vi "AUTO - REVERSE from DASHB.vi"() -> ()   [LabVIEW 2020]
uses:
  Robot Global Data.vi
  <vilib>/Rock Robotics/Network Tables/NT Write Boolean.vi
  <vilib>/Rock Robotics/WPI/Utilities/WPI_GetSetVariantRefNum.vi
  <vilib>/Rock Robotics/Network Tables/NT Read Number.vi
  <vilib>/Rock Robotics/Network Tables/NT Read Boolean.vi
  <vilib>/Rock Robotics/Network Tables/NT Write Number.vi
panel:
  out "time drive (s)":dbl
  out "SHOOTER %PREV":dbl
  in  "NT stack ref":string="AUTO SET/"
  out "motor command":dbl
  out "motor run time (s)":dbl
  out "distance (in)":dbl
  out "free velocity (in/s)":dbl
  out "throttle":dbl
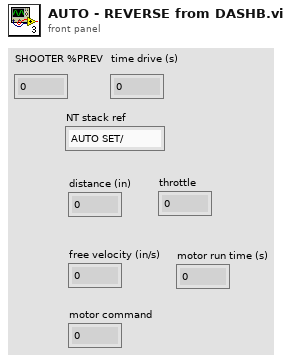
[diagram p1: front panel]
types:
  T1 = cluster{"DRIVE gear ratio":dbl, "DRIVE wheel diameter (in)":dbl, "DRIVE free speed rpm":dbl, "DRIVE min output":dbl, "DRIVE stall in-lbf":dbl}
  T2 = typedef "WPI_RobotDriveDevRef.ctl" = cluster{"DevStatus":errorcluster, "Motors[]":T3[], "Square Inputs":bool, "Max Output":dbl}
  T3 = typedef "WPI_MotorControlDeviceRef.ctl" = cluster{"DeviceStatus":errorcluster, "Type":T4, "PWM":cluster{"PWM Channel":T5, "DeadBand":T6}, "CAN":cluster{"Device Number":u8, "SetOutput VI Ref":variant, "GetOutput VI Ref":variant, "Enable VI Ref":variant, "Disable VI Ref":variant, "Data":variant}, "Invert":bool, "DIO PWM":cluster{"PWM \"Enable\" Channel":T5, "DIOChannel":T7, "PWM Rate":dbl}}
  T4 = typedef "WPI_MotorControlType.ctl" = enum16{"PWM", "CAN", "DIO PWM"}
  T5 = typedef "FPGA_DIOPWMChannel.ctl" = enum8{"PWM 0", "PWM 1", "PWM 2", "PWM 3", "PWM 4", "PWM 5", "PWM 6", "PWM 7", "PWM 8", "PWM 9", "PWM MXP 0", "PWM MXP 1", "PWM MXP 2", "PWM MXP 3", "PWM MXP 4", "PWM MXP 5", "PWM MXP 6", "PWM MXP 7", "PWM MXP 8", "PWM MXP 9", "Invalid"}
  T6 = typedef "WPI_PWMDeadband.ctl" = cluster{"Name":string, "maxPositivePwm":i32, "minPositivePwm":i32, "centerPwm":i32, "maxNegativePwm":i32, "minNegativePwm":i32, "angularRange":u16}
  T7 = typedef "FPGA_DIOChannel.ctl" = enum8{"DIO 0", "DIO 1", "DIO 2", "DIO 3", "DIO 4", "DIO 5", "DIO 6", "DIO 7", "DIO 8", "DIO 9", "DIO MXP 0", "DIO MXP 1", "DIO MXP 2", "DIO MXP 3", "DIO MXP 4", "DIO MXP 5", "DIO MXP 6", "DIO MXP 7", "DIO MXP 8", "DIO MXP 9", "DIO MXP 10", "DIO MXP 11", "DIO MXP 12", "DIO MXP 13", "DIO MXP 14", "DIO MXP 15", "SPI Port CS1", "SPI Port CS2", "SPI Port CS3", "SPI Port MISO", "SPI Port MOSI", "Invalid"}
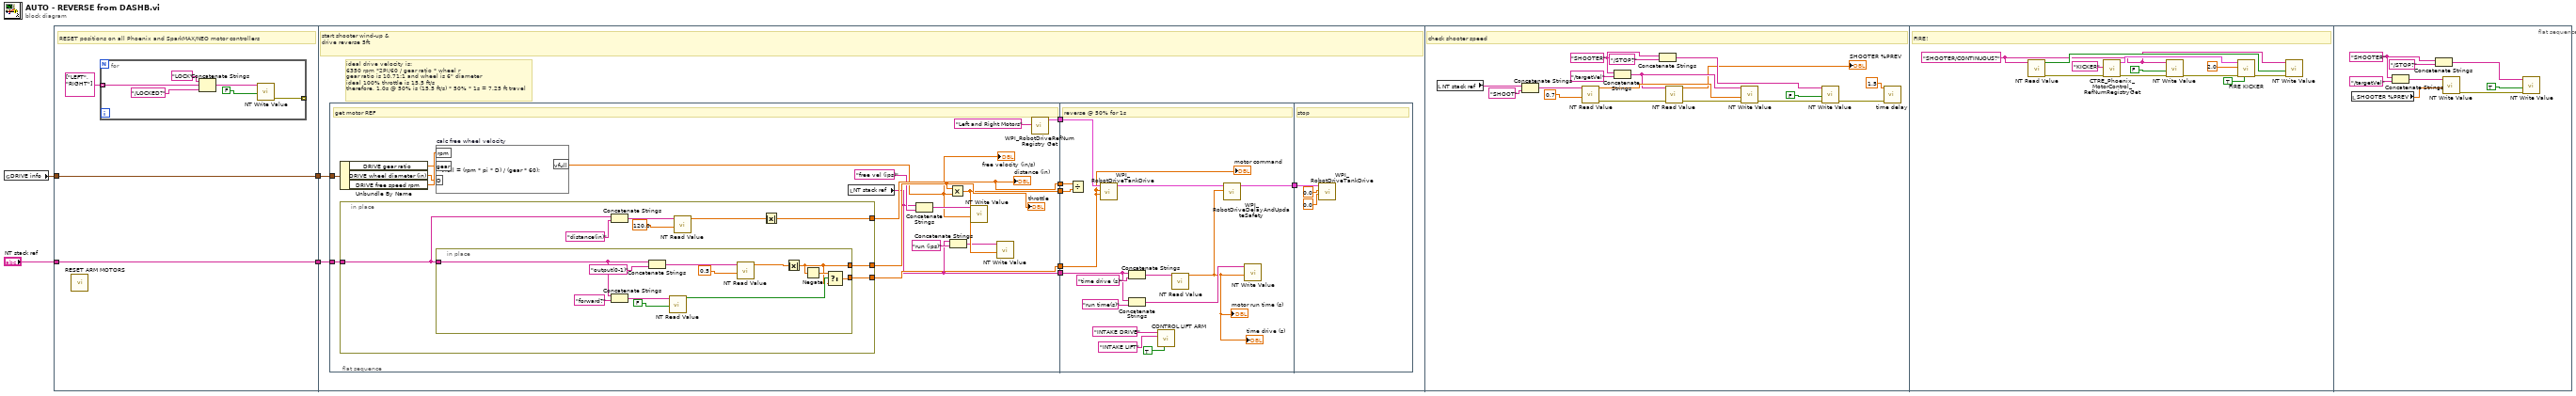
[diagram p0: block diagram]
diagram:
  n1 = global read "Robot Global Data.vi" "DRIVE info"() -> (w4:T1)
  n2 = flat-sequence {
    tunnel: w4 -> [w6]
    tunnel: [w6] -> w2
    tunnel: "NT stack ref" -> [w5]
    tunnel: [w5] -> w1
    tunnel: w2 -> [w15]
    tunnel: w1 -> [w14]
    frame #0 {
      # "RESET positions on all Phoenix and SparkMAX/NEO motor controllers"
      n3 = call "RESET ARM MOTORS.vi"() -> ()  [unwired: 9 in, 3 out]
      n4 = for {
        tunnel: string[] ["LEFT", "RIGHT"] -> [w10] mode=indexing
        tunnel: [w8] -> _ mode=indexing
        n5 = Concatenate Strings("LOCK" ("string"), w10, "/LOCKED?" ("Name")) -> (w12:string)
        n6 = call-poly <vilib>:"NT Write Value.vi"("Boolean"=FALSE, "Name"=w12) -> ("error out"=w8:errorcluster)  [unwired: 9 in]
      }
    }
    frame #1 {
      # "ideal drive velocity is:\n6350 rpm *2PI/60 / gear ratio * wheel r\ngear ratio is 10.71:1 and wheel is 6\" diameter\nideal 100% throttle is 15.5 ft/s\ntherefore, 1.0s @ 50% is (15.5 ft/s) * 50% * 1s = 7.25 ft travel"
      # "start shooter wind-up &\ndrive reverse 5ft"
      n7 = flat-sequence {
        tunnel: [w37] -> w21
        tunnel: w15 -> [w36]
        tunnel: w14 -> [w32]
        tunnel: [w31] -> w19
        tunnel: [w30] -> w18
        tunnel: [w25] -> w17
        tunnel: [w22] -> w16
        tunnel: w21 -> [w72]
        tunnel: [w71] -> w20
        tunnel: w19 -> [w70]
        tunnel: w18 -> [w69]
        tunnel: w17 -> [w68]
        tunnel: w16 -> [w63]
        tunnel: w20 -> [w74]
        frame #0 {
          # "get motor REF"
          n8 = Unbundle By Name(w36) -> ("DRIVE gear ratio"=w34:dbl, "DRIVE wheel diameter (in)"=w33:dbl, "DRIVE free speed rpm"=w35:dbl)
          n9 = in-place {
            in-place-border: w32 -> [w42]
            in-place-border: [w41] -> w31
            in-place-border: [w40] -> w30
            in-place-border: [w39] -> w29
            n10 = in-place {
              in-place-border: w42 -> [w50]
              in-place-border: [w49] -> w41
              in-place-border: [w47] -> w39
              n11 = Concatenate Strings(w50, "forward?" ("string")) -> (w54:string)
              n12 = Concatenate Strings(w50, "output(0-1)" ("string")) -> (w58:string)
              n13 = call-poly <vilib>:"NT Read Value.vi"("Default Value"=FALSE, "Name"=w54) -> ("Boolean"=w52:bool)  [unwired: 8 in, 1 out]
              n14 = call-poly <vilib>:"NT Read Value.vi"("Default Value"=0.5, "Name"=w58) -> ("Numeric"=w55:dbl)  [unwired: 8 in, 1 out]
              n15 = Absolute Value(x=w55) -> (abs(x)=w47:dbl)
              n16 = Negate(x=w47) -> (-x=w51:dbl)
              n17 = Select(t=w51, s=w52, f=w47) -> (s? t:f=w49:dbl)
            }
            n18 = Concatenate Strings(w42, "distance(in)" ("string")) -> (w46:string)
            n19 = call-poly <vilib>:"NT Read Value.vi"("Default Value"=120.0, "Name"=w46) -> ("Numeric"=w43:dbl)  [unwired: 8 in, 1 out]
            n20 = Absolute Value(x=w43) -> (abs(x)=w40:dbl)
          }
          "distance (in)" <- w30
          "throttle" <- w29
          n21 = formula code="vfull = (rpm * pi * D) / (gear * 60);" "calc free wheel velocity"("rpm"=w35, "gear"=w34, "D"=w33) -> ("vfull"=w26:dbl)
          "free velocity (in/s)" <- w26
          n22 = local read "NT stack ref"() -> (w22:string)
          n23 = Concatenate Strings(w22, "free vel (ips)" ("string")) -> (w28:string)
          n24 = Multiply(x=w29, y=w26) -> (x*y=w25:dbl)
          n25 = Concatenate Strings(w22, "run (ips)" ("string")) -> (w24:string)
          n26 = call-poly <vilib>:"NT Write Value.vi"("Numeric"=w26, "Name"=w28) -> ()  [unwired: 9 in, 1 out]
          n27 = call-poly <vilib>:"NT Write Value.vi"("Numeric"=w25, "Name"=w24) -> ()  [unwired: 9 in, 1 out]
          n28 = call <vilib>:"WPI_RobotDriveRefNum Registry Get.vi"("refnum name"="Left and Right Motors") -> ("RobotDriveDevRef"=w37:T2)  [unwired: 1 in, 9 out]
        }
        frame #1 {
          # "reverse @ 50% for 1s"
          n29 = Divide(x=w69, y=w68) -> ()  [unwired: 1 out]
          n30 = call <vilib>:"WPI_RobotDriveTankDrive.vi"("Right axis value"=w70, "Left axis value"=w70, "RobotDriveDevRef"=w72) -> ("RobotDriveDevRef"=w73:T2)  [unwired: 6 in, 2 out]
          n31 = Concatenate Strings(w63, "time drive (s)" ("string")) -> (w65:string)
          n32 = Concatenate Strings(w63, "run time(s)" ("string")) -> (w67:string)
          n33 = call "CONTROL LIFT ARM.vi"("force extend?"=TRUE, "LIFT ARM refname"="INTAKE LIFT", "LIFT DRIVE refname"="INTAKE DRIVE") -> ()  [unwired: 8 in, 1 out]
          n34 = call-poly <vilib>:"NT Read Value.vi"("Name"=w65) -> ("Numeric"=w62:dbl)  [unwired: 9 in, 1 out]
          "motor run time (s)" <- w62
          "time drive (s)" <- w62
          n35 = call <vilib>:"WPI_RobotDriveDelayAndUpdateSafety.vi"("Delay (s)"=w62, "RobotDriveDevRef"=w73) -> ("RobotDriveDevRef 2"=w71:T2)  [unwired: 8 in, 1 out]
          n36 = call-poly <vilib>:"NT Write Value.vi"("Numeric"=w62, "Name"=w67) -> ()  [unwired: 9 in, 1 out]
          "motor command" <- w70
        }
        frame #2 {
          # "stop"
          n37 = call <vilib>:"WPI_RobotDriveTankDrive.vi"("Right axis value"=0.0 ("X axis value"), "Left axis value"=0.0 ("X axis value"), "RobotDriveDevRef"=w74) -> ()  [unwired: 6 in, 3 out]
        }
      }
    }
    frame #2 {
      w92 = "SHOOTER" ("Name")
      # "check shooter speed"
      n38 = local read "NT stack ref"() -> (w84:string)
      n39 = Concatenate Strings(w84, "SHOOT") -> (w83:string)
      n40 = call-poly <vilib>:"NT Read Value.vi"("Default Value"=0.7, "Name"=w83) -> ("error out"=w79:errorcluster, "Numeric"=w82:dbl)  [unwired: 8 in]
      n41 = Concatenate Strings(w92, "/targetVel" ("Name")) -> (w80:string)
      n42 = Concatenate Strings(w92, "/STOP?" ("string")) -> (w91:string)
      n43 = call-poly <vilib>:"NT Read Value.vi"("error in"=w79, "Name"=w80) -> ("error out"=w78:errorcluster, "Numeric"=→"SHOOTER %PREV":dbl)  [unwired: 8 in]
      n44 = call-poly <vilib>:"NT Write Value.vi"("error in"=w78, "Numeric"=w82, "Name"=w80) -> ("error out"=w88:errorcluster)  [unwired: 8 in]
      n45 = call-poly <vilib>:"NT Write Value.vi"("error in"=w88, "Boolean"=FALSE, "Name"=w91) -> ("error out"=w87:errorcluster)  [unwired: 8 in]
      n46 = call "time delay.vi"("error in (no error)"=w87, "timer delay (s)"=1.5) -> ()  [unwired: 8 in, 2 out]
    }
    frame #3 {
      w94 = "SHOOTER/CONTINUOUS?" ("Name")
      # "FIRE!"
      n47 = call-poly <vilib>:"NT Read Value.vi"("Name"=w94) -> ("error out"=w97:errorcluster, "Boolean"=w95:bool)  [unwired: 9 in]
      n48 = call <vilib>:"CTRE_Phoenix_MotorControl_RefNumRegistryGet.vi"("error in (no error)"=w97, "refnum name"="KICKER") -> ("error out"=w98:errorcluster, "PhoenixMotorControlDevRef"=w99:T3)  [unwired: 8 in]
      n49 = call-poly <vilib>:"NT Write Value.vi"("error in"=w98, "Boolean"=FALSE, "Name"=w94) -> ("error out"=w101:errorcluster)  [unwired: 8 in]
      n50 = call "FIRE KICKER.vi"("force fire?"=TRUE, "error in (no error)"=w101, "delay seconds"=2.0, "VictorSPX devref in"=w99) -> ("error out"=w96:errorcluster)  [unwired: 6 in, 1 out]
      n51 = call-poly <vilib>:"NT Write Value.vi"("error in"=w96, "Boolean"=w95, "Name"=w94) -> ()  [unwired: 8 in, 1 out]
    }
    frame #4 {
      w110 = "SHOOTER" ("Name")
      n52 = local read "SHOOTER %PREV"() -> (w105:dbl)
      n53 = Concatenate Strings(w110, "/targetVel" ("Name")) -> (w112:string)
      n54 = Concatenate Strings(w110, "/STOP?" ("string")) -> (w109:string)
      n55 = call-poly <vilib>:"NT Write Value.vi"("Numeric"=w105, "Name"=w112) -> ("error out"=w106:errorcluster)  [unwired: 9 in]
      n56 = call-poly <vilib>:"NT Write Value.vi"("error in"=w106, "Boolean"=TRUE, "Name"=w109) -> ()  [unwired: 8 in, 1 out]
    }
  }
